vi "rqcBob Serch for Supported HW.vi"(8 "error in":errorcluster, 11 "Expected Resource Name":string) -> (0 "error out":errorcluster, 2 "Compatible Devices List":string[][](array[string]))   [LabVIEW 2019, in "rqcBob.lvclass"]
uses:
  rqcBob.lvclass
  <vilib>/nisyscfg/Filter Mode.ctl
  <vilib>/nisyscfg/Close (Hardware).vi
  <vilib>/nisyscfg/Close (Filter).vi
  <vilib>/nisyscfg/Close (System).vi
  <vilib>/nisyscfg/nisyscfg.lvlib
  <resource>/objmgr/nisysapi.rc
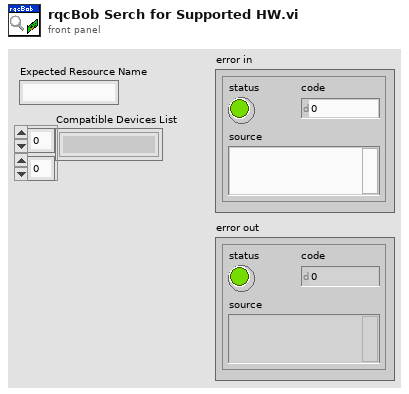
[diagram p1: front panel]
types:
  T1 = typedef "nisyscfg.lvlib/Filter Mode.ctl" = i32
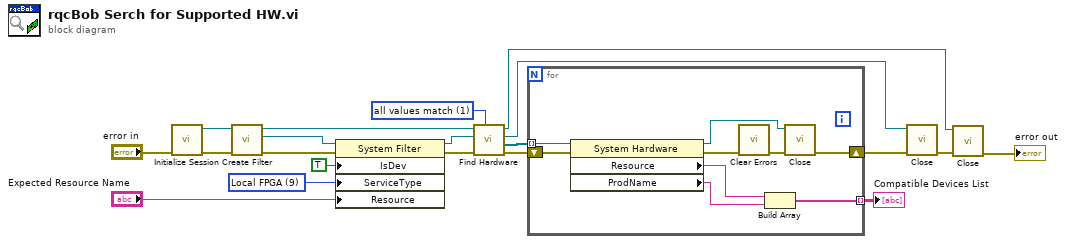
[diagram p0: block diagram]
diagram:
  w11 = T1 1 items=["all values match"=1, "any value matches"=2, "values do not match"=3, "all properties exist"=4] ("Filter Mode (all values match)")
  w15 = u32 9 items=["NI Network Resource", "NI Real-Time", "NI System Configuration", "NI Web Interface", "Local System", "Local Network Adapter", "Local Time Keeper", "Local Time Reference", "LXI Instrument", "Local FPGA"] ("Service Type")
  n1 = call <vilib>:"Initialize Session.vi"("error in (no error)"="error in") -> ("error out"=w17:errorcluster, "Session out"=w18:refnum<k21>)  [unwired: 9 in]
  n2 = call <vilib>:"Create Filter.vi"("error in (no error)"=w17, "Session in"=w18) -> ("error out"=w20:errorcluster, "Filter out"=w19:refnum<k20>, "Session out"=w14:refnum<k21>)  [unwired: 7 in]
  n3 = property class="System Filter"(reference=w19, error in=w20, "IsDev"=TRUE ("Is Device"), "ServiceType"=w15, "Resource"="Expected Resource Name") -> (reference out=w12:refnum<k20>, error out=w13:errorcluster)
  n4 = call <vilib>:"Find Hardware.vi"("Filter Mode (all values match)"=w11, "error in (no error)"=w13, "Filter in"=w12, "Session in"=w14) -> ("error out"=w10:errorcluster, "Resources out"=w9:refnum<k20>[], "Filter out"=w7:refnum<k20>, "Session out"=w5:refnum<k21>)  [unwired: 4 in]
  n5 = for {
    shift-right: [w24] -> w8
    shift-left: w10 -> [w26]
    tunnel: w9 -> [w29] mode=indexing
    tunnel: [w21] -> w1 mode=indexing
    n6 = property class="System Hardware"(reference=w29, error in=w26) -> (reference out=w28:refnum<k20>, error out=w27:errorcluster, "Resource"=w23:string, "ProdName"=w22:string)
    n7 = call <vilib>:"Clear Errors.vi"("error in (no error)"=w27) -> ("error out"=w25:errorcluster)  [unwired: 5 in, 1 out]
    n8 = Build Array(w23, w22) -> (w21:string[])
    n9 = call-poly <vilib>:"Close.vi"("error in (no error)"=w25, "Resource in"=w28) -> ("error out"=w24:errorcluster)  [unwired: 9 in]
  }
  "Compatible Devices List" <- w1
  n10 = call-poly <vilib>:"Close.vi"("error in (no error)"=w8, "Filter in"=w7) -> ("error out"=w6:errorcluster)  [unwired: 9 in]
  n11 = call-poly <vilib>:"Close.vi"("error in (no error)"=w6, "Session in"=w5) -> ("error out"=→"error out":errorcluster)  [unwired: 9 in]
